vi "Write Variant Page Data.vi"(0 "Byte Stream File in":refnum<file>, 2 "Details":T2 {"PhotometricInterpretation" items=["MIN IS WHITE"=0, "MIN IS BLACK"=1, "RGB"=2, "PALETTE"=3, "MASK"=4, "SEPARATED"=5, "YCBCR"=6, "CIE LAB"=8, "ICC LAB"=9, "ITU LAB"=10, "LOGL"=32844, "LOGLUV"=32845, "CFA"=32803, "LinearRaw"=34892, "DEPTH"=51177]}, 5 "byte order (0:big-endian, network order)":T3(ring), 9 "Image Data":variant, 11 "error in (no error)":errorcluster, 13 "Settings":T1={"zlib compression level"=-1, "Max Strip bytes"=8192, "JPEG Quality (85)"=85}) -> (1 "Size(s)":u32[](array[numeric]), 3 "Bits per Sample":u32, 4 "Byte Stream File out":refnum<file>, 6 "Signed":bool, 8 "Data Bytes":i64, 10 "Bytes Per Sample":u32, 12 "Fractional":bool, 14 "Samples Per Pixel":i32, 15 "error out":errorcluster)   [LabVIEW 2020, in "LV Tiff.lvlib"]
uses:
  LV Tiff.lvlib
  Tiff Page Details.ctl
  Page Writer Settings.ctl
  <vilib>/picture/picture.llb/imagedata.ctl
  <vilib>/Utility/Data Type/NI_Data Type.lvlib
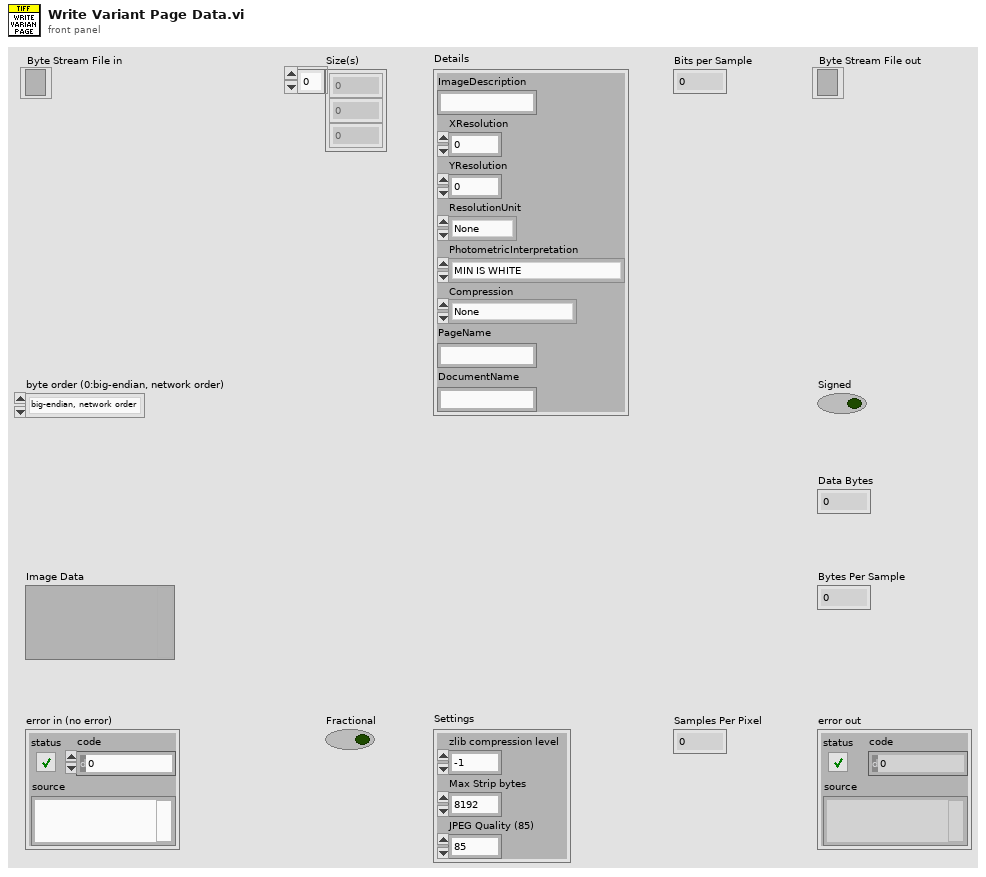
[diagram p1: front panel]
types:
  T1 = typedef "LV Tiff.lvlib/Page Writer Settings.ctl" = cluster{"zlib compression level":i32, "Max Strip bytes":u32, "JPEG Quality (85)":i32}
  T2 = typedef "LV Tiff.lvlib/Tiff Page Details.ctl" = cluster{"ImageDescription":string, "XResolution":dbl, "YResolution":dbl, "ResolutionUnit":enum16{"None", "Inch", "Centimeter"}, "PhotometricInterpretation":u16, "Compression":enum16{"None", "Deflate", "JPEG"}, "PageName":string, "DocumentName":string}
  T3 = enum16{"big-endian, network order", "native, host order", "little-endian"}
  T4 = typedef "imagedata.ctl" = cluster{"image type":i32, "image depth":i32, "image":u8[], "mask":u8[], "colors":u32[], "Rectangle":cluster{"left":i16, "top":i16, "right":i16, "bottom":i16}}
  T5 = typedef "NI_Data Type.lvlib/Data Type.ctl" = enum8{"Invalid Type", "Void", "I8", "I16", "I32", "I64", "U8", "U16", "U32", "U64", "Single Float", "Double Float", "Extended Float", "Single Complex", "Double Complex", "Extended Complex", "Enum U8", "Enum U16", "Enum U32", "Enum U64", "Single Float With Unit", "Double Float With Unit", "Extended Float With Unit", "Single Complex with Unit", "Double Complex with Unit", "Extended Complex with Unit", "Boolean", "String", "Path", "Picture", "Tag", "Array", "Cluster", "Variant", "LV Variant", "Waveform", "Timestamp", "Digital Waveform", "Digital Data", "ExpressData", "Refnum", "External Data", "VI", "Poly VI", "LabVIEW Class Instance", "Fixed Point", "Set Collection", "Map Collection"}
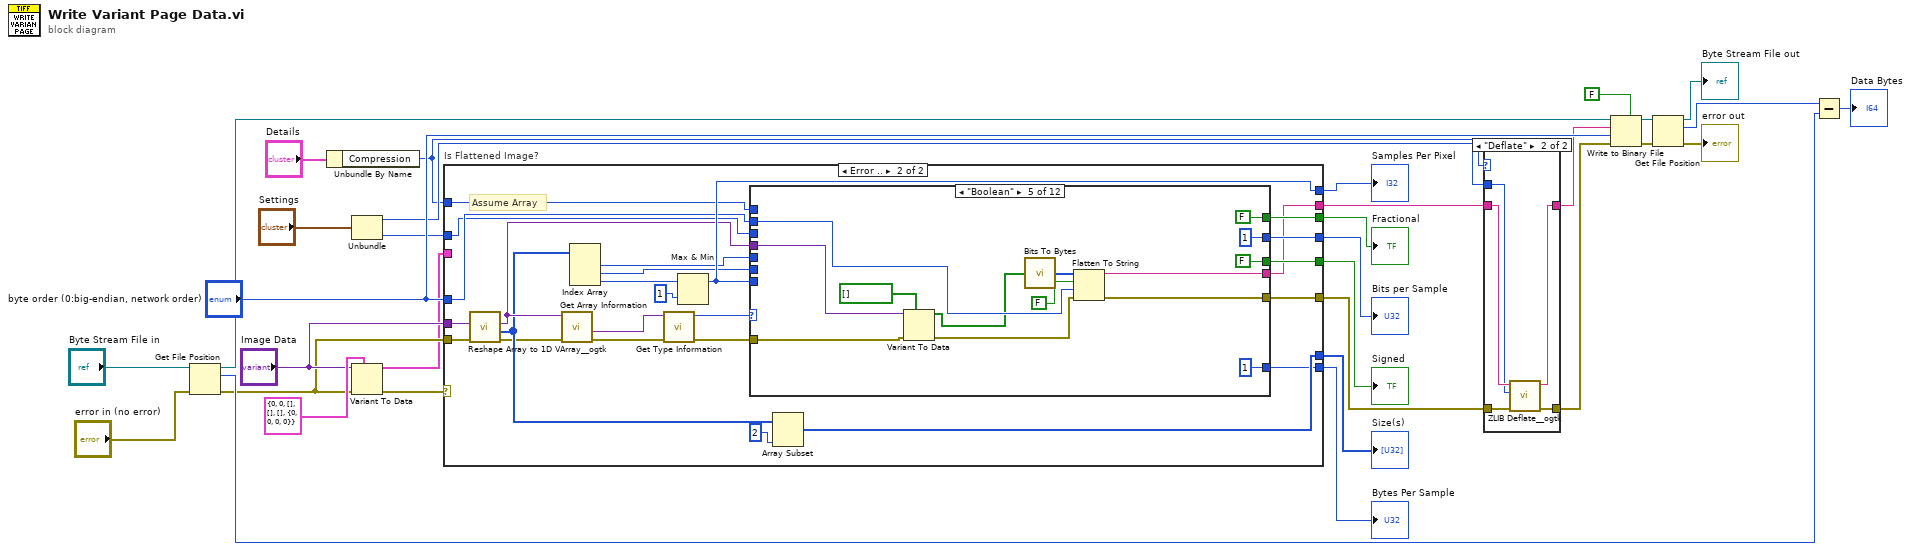
[diagram p0: block diagram]
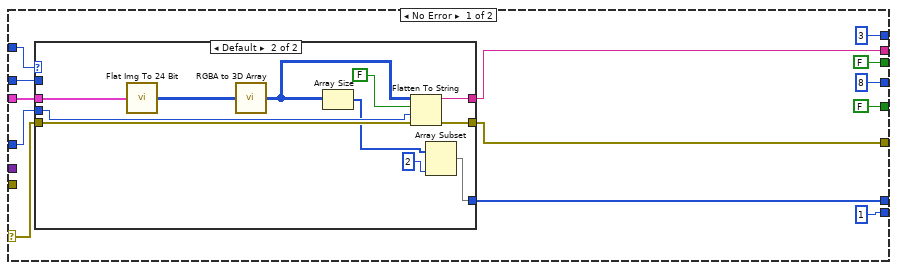
[diagram p2: hidden frame]
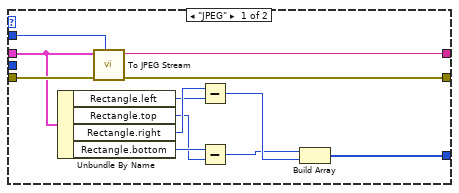
[diagram p3: hidden frame]
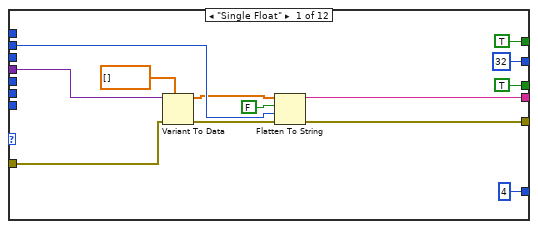
[diagram p4: hidden frame]
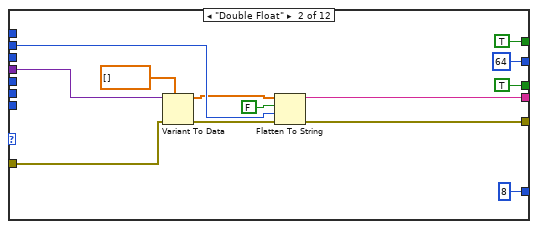
[diagram p5: hidden frame]
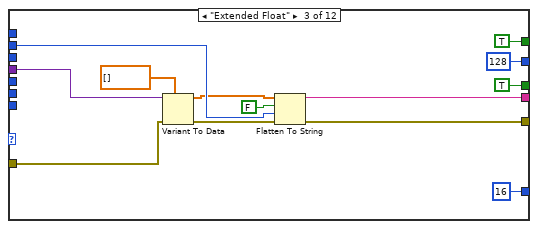
[diagram p6: hidden frame]
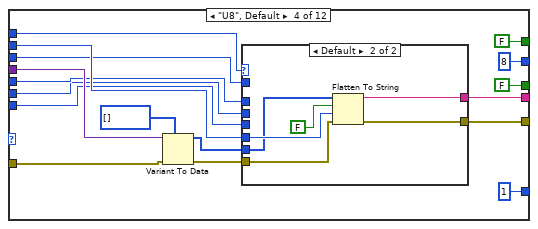
[diagram p7: hidden frame]
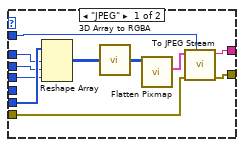
[diagram p8: hidden frame]
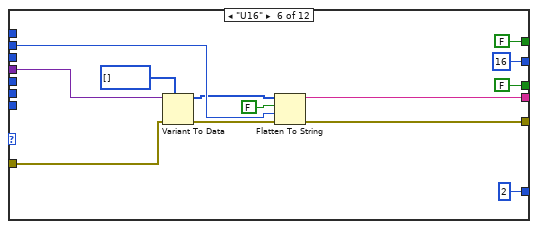
[diagram p9: hidden frame]
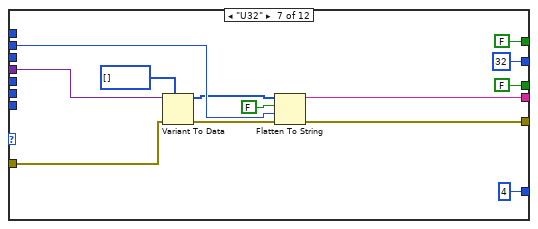
[diagram p10: hidden frame]
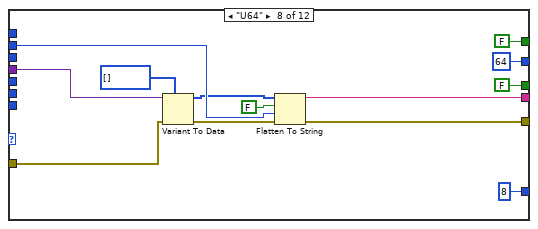
[diagram p11: hidden frame]
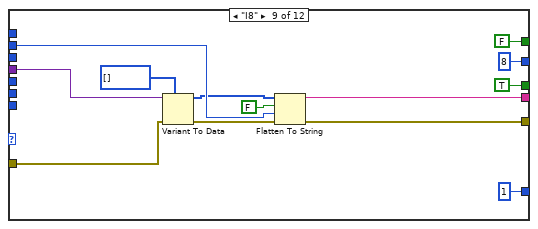
[diagram p12: hidden frame]
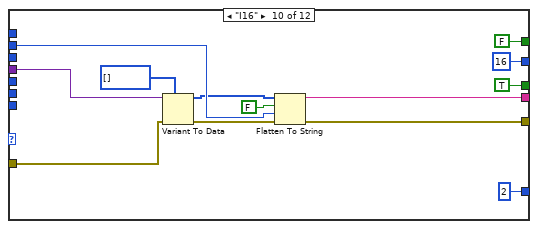
[diagram p13: hidden frame]
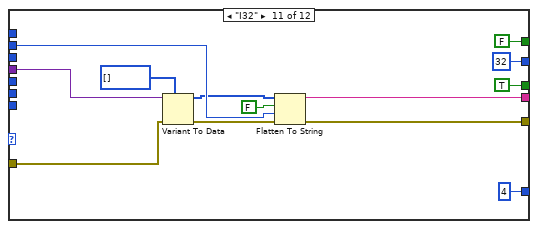
[diagram p14: hidden frame]
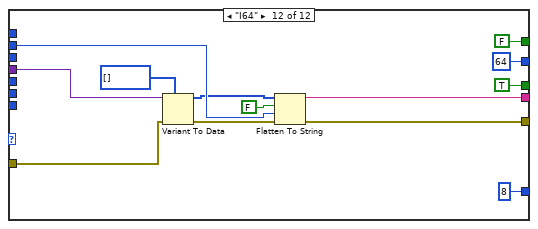
[diagram p15: hidden frame]
diagram:
  n1 = Get File Position(4:"error in (no error)", 7:"Byte Stream File in") -> (0:w4:errorcluster, 2:w17:i64, 3:w19:refnum<file>)
  n2 = Unbundle By Name("Details") -> ("Compression"=w7:enum16{"None", "Deflate", "JPEG"})
  n3 = Unbundle("Settings") -> ("zlib compression level"=w8:i32, "JPEG Quality (85)"=w1:i32)  [unwired: 1 out]
  n4 = Variant To Data(error in=w4, type=T4 {"image type"=0, "image depth"=0, "image"=[], "mask"=[], "colors"=[], "Rectangle"={"left"=0, "top"=0, "right"=0, "bottom"=0}} ("image data"), Variant="Image Data") -> (data=w2:T4, error out=w3:errorcluster)
  n5 = case "Is Flattened Image?" shown="Error .." w3 {
    selector: w3 -> [w38 _]
    tunnel: [u32 3 w93] -> w32
    tunnel: [w35 w92] -> w30
    tunnel: [u32 8 w91] -> w29
    tunnel: [u32 1 w90] -> w28
    tunnel: [FALSE w89] -> w27
    tunnel: [FALSE w88] -> w26
    tunnel: "byte order (0:big-endian, network order)" -> [w39 w87]
    tunnel: w4 -> [_ w74]
    tunnel: [w36 w73] -> w13
    tunnel: [w37 w72] -> w12
    tunnel: w7 -> [w34 w71]
    tunnel: "Image Data" -> [_ w70]
    tunnel: w2 -> [w40 _]
    tunnel: w1 -> [w33 w69]
    frame No Error {
      n6 = case shown="Default" w34 {
        tunnel: w40 -> [w54 w68]
        tunnel: w39 -> [_ w67]
        tunnel: w38 -> [w57 w66]
        tunnel: [w55 w65] -> w37
        tunnel: [w56 w64] -> w36
        tunnel: [w47 w59] -> w35
        tunnel: w33 -> [w46 _]
        frame "JPEG" {
          n7 = Unbundle By Name(w54) -> ("Rectangle.left"=w52:i16, "Rectangle.top"=w50:i16, "Rectangle.right"=w53:i16, "Rectangle.bottom"=w51:i16)
          n8 = call "To JPEG Stream.vi"("Quality (85)"=w46, "error out"=w57, "image data"=w54) -> ("error out"=w56:errorcluster, "data"=w55:string)  [unwired: 7 in]
          n9 = Subtract(x=w53, y=w52) -> (x-y=w49:i16)
          n10 = Subtract(x=w51, y=w50) -> (x-y=w48:i16)
          n11 = Build Array(w48, w49) -> (w47:i16[])
        }
        frame Default {
          n12 = call "Flat Img To 24 Bit.vi"("image data"=w68) -> ("24-bit pixmap"=w62:u32[][])
          n13 = call "RGBA to 3D Array.vi"("24-bit pixmap"=w62) -> ("RGB Array"=w60:u8[][][])  [unwired: 1 in]
          n14 = Array Size(array=w60) -> (size(s)=w61:i32[])
          n15 = Flatten To String(anything=w60, prepend array or string size? (T)=FALSE, byte order (0:big-endian, network order)=w67, error in (no error)=w66) -> (data string=w65:string, error out=w64:errorcluster)  [unwired: 1 out]
          n16 = Array Subset(array=w61, length=2) -> (w59:i32[])  [unwired: 1 in]
        }
      }
    }
    frame Error {
      # "Assume Array"
      n17 = call <userlib>:"Reshape Array to 1D VArray__ogtk.vi"("error in (no error)"=w74, "MultiD Array"=w70) -> ("error out"=w78:errorcluster, "Size(s)"=w80:u32[], "1D VArray"=w82:variant)  [unwired: 7 in]
      n18 = call <vilib>:"Get Array Information.vi"("error in (no error)"=w78, "variant"=w82) -> ("error out"=w84:errorcluster, "array element data type"=w83:variant)  [unwired: 6 in, 2 out]
      n19 = Index Array(array=w80) -> (element #1=w76:u32, element #2=w75:u32, element #3=w77:u32)  [unwired: 3 in]
      n20 = call <vilib>:"Get Type Information.vi"("error in (no error)"=w84, "variant"=w83) -> ("error out"=w86:errorcluster, "type"=w85:T5)  [unwired: 5 in, 3 out]
      n21 = Max & Min(x=w77, y=u32 1) -> (max(x,y)=w93:u32)  [unwired: 1 out]
      n22 = case shown="\"Boolean\"" w85 {
        tunnel: w87 -> [w105 w118 w131 w148 w179 w192 w205 w218 w231 w244 w257 w270]
        tunnel: [w104 w117 w130 w149 w180 w191 w204 w217 w230 w243 w256 w269] -> w73
        tunnel: [TRUE ("Signed") TRUE ("Signed") TRUE ("Signed") FALSE ("Signed") FALSE ("Signed") FALSE ("Signed") FALSE ("Signed") FALSE ("Signed") TRUE ("Signed") TRUE ("Signed") TRUE ("Signed") TRUE ("Signed")] -> w88
        tunnel: [TRUE ("Fractional") TRUE ("Fractional") TRUE ("Fractional") FALSE ("Fractional") FALSE ("Fractional") FALSE ("Fractional") FALSE ("Fractional") FALSE ("Fractional") FALSE ("Fractional") FALSE ("Fractional") FALSE ("Fractional") FALSE ("Fractional")] -> w89
        tunnel: [4 ("#Bytes") 8 ("#Bytes") 16 ("#Bytes") 1 ("#Bytes") 1 ("#Bytes") 2 ("#Bytes") 4 ("#Bytes") 8 ("#Bytes") 1 ("#Bytes") 2 ("#Bytes") 4 ("#Bytes") 8 ("#Bytes")] -> w90
        tunnel: [32 ("# Bits") 64 ("# Bits") 128 ("# Bits") 8 ("# Bits") 1 ("# Bits") 16 ("# Bits") 32 ("# Bits") 64 ("# Bits") 8 ("# Bits") 16 ("# Bits") 32 ("# Bits") 64 ("# Bits")] -> w91
        tunnel: w86 -> [w103 w116 w129 w145 w177 w190 w203 w216 w229 w242 w255 w268]
        tunnel: w82 -> [w102 w115 w128 w144 w176 w189 w202 w215 w228 w241 w254 w267]
        tunnel: w76 -> [_ _ _ w140 _ _ _ _ _ _ _ _]
        tunnel: w75 -> [_ _ _ w139 _ _ _ _ _ _ _ _]
        tunnel: w93 -> [_ _ _ w138 _ _ _ _ _ _ _ _]
        tunnel: [w94 w107 w120 w147 w178 w181 w194 w207 w220 w233 w246 w259] -> w72
        tunnel: w71 -> [_ _ _ w146 _ _ _ _ _ _ _ _]
        tunnel: w69 -> [_ _ _ w133 _ _ _ _ _ _ _ _]
        frame "Single Float" {
          n23 = Variant To Data(error in=w103, type=sgl[] [], Variant=w102) -> (data=w95:sgl[], error out=w100:errorcluster)
          n24 = Flatten To String(anything=w95, prepend array or string size? (T)=FALSE, byte order (0:big-endian, network order)=w105, error in (no error)=w100) -> (data string=w94:string, error out=w104:errorcluster)  [unwired: 1 out]
        }
        frame "Double Float" {
          n25 = Variant To Data(error in=w116, type=dbl[] [], Variant=w115) -> (data=w113:dbl[], error out=w112:errorcluster)
          n26 = Flatten To String(anything=w113, prepend array or string size? (T)=FALSE, byte order (0:big-endian, network order)=w118, error in (no error)=w112) -> (data string=w107:string, error out=w117:errorcluster)  [unwired: 1 out]
        }
        frame "Extended Float" {
          n27 = Variant To Data(error in=w129, type=ext[] [], Variant=w128) -> (data=w126:ext[], error out=w125:errorcluster)
          n28 = Flatten To String(anything=w126, prepend array or string size? (T)=FALSE, byte order (0:big-endian, network order)=w131, error in (no error)=w125) -> (data string=w120:string, error out=w130:errorcluster)  [unwired: 1 out]
        }
        frame "U8", Default {
          n29 = Variant To Data(error in=w145, type=u8[] [], Variant=w144) -> (data=w141:u8[], error out=w142:errorcluster)
          n30 = case shown="Default" w146 {
            tunnel: [w152 w166] -> w149
            tunnel: w148 -> [_ w165]
            tunnel: [w151 w163] -> w147
            tunnel: w142 -> [w153 w162]
            tunnel: w141 -> [w160 w161]
            tunnel: w140 -> [w159 _]
            tunnel: w139 -> [w158 _]
            tunnel: w138 -> [w157 _]
            tunnel: w133 -> [w150 _]
            frame "JPEG" {
              n31 = Reshape Array(w160, w159, w158, w157) -> (w156:u8[][][])
              n32 = call "3D Array to RGBA.vi"("3D Array"=w156) -> ("RGBA"=w155:u32[][])
              n33 = call <vilib>:"Flatten Pixmap.vi"("24-bit pixmap"=w155) -> ("image data"=w154:T4)  [unwired: 10 in]
              n34 = call "To JPEG Stream.vi"("Quality (85)"=w150, "error out"=w153, "image data"=w154) -> ("error out"=w152:errorcluster, "data"=w151:string)  [unwired: 7 in]
            }
            frame Default {
              n35 = Flatten To String(anything=w161, prepend array or string size? (T)=FALSE, byte order (0:big-endian, network order)=w165, error in (no error)=w162) -> (data string=w163:string, error out=w166:errorcluster)  [unwired: 1 out]
            }
          }
        }
        frame "Boolean" {
          n36 = Variant To Data(error in=w177, type=bool[] [], Variant=w176) -> (data=w173:bool[], error out=w174:errorcluster)
          n37 = call "Bits To Bytes.vi"("Bits"=w173) -> ("Bytes"=w167:u8[])
          n38 = Flatten To String(anything=w167, prepend array or string size? (T)=FALSE, byte order (0:big-endian, network order)=w179, error in (no error)=w174) -> (data string=w178:string, error out=w180:errorcluster)  [unwired: 1 out]
        }
        frame "U16" {
          n39 = Variant To Data(error in=w190, type=u16[] [], Variant=w189) -> (data=w187:u16[], error out=w186:errorcluster)
          n40 = Flatten To String(anything=w187, prepend array or string size? (T)=FALSE, byte order (0:big-endian, network order)=w192, error in (no error)=w186) -> (data string=w181:string, error out=w191:errorcluster)  [unwired: 1 out]
        }
        frame "U32" {
          n41 = Variant To Data(error in=w203, type=u32[] [], Variant=w202) -> (data=w200:u32[], error out=w199:errorcluster)
          n42 = Flatten To String(anything=w200, prepend array or string size? (T)=FALSE, byte order (0:big-endian, network order)=w205, error in (no error)=w199) -> (data string=w194:string, error out=w204:errorcluster)  [unwired: 1 out]
        }
        frame "U64" {
          n43 = Variant To Data(error in=w216, type=u64[] [], Variant=w215) -> (data=w213:u64[], error out=w212:errorcluster)
          n44 = Flatten To String(anything=w213, prepend array or string size? (T)=FALSE, byte order (0:big-endian, network order)=w218, error in (no error)=w212) -> (data string=w207:string, error out=w217:errorcluster)  [unwired: 1 out]
        }
        frame "I8" {
          n45 = Variant To Data(error in=w229, type=i8[] [], Variant=w228) -> (data=w226:i8[], error out=w225:errorcluster)
          n46 = Flatten To String(anything=w226, prepend array or string size? (T)=FALSE, byte order (0:big-endian, network order)=w231, error in (no error)=w225) -> (data string=w220:string, error out=w230:errorcluster)  [unwired: 1 out]
        }
        frame "I16" {
          n47 = Variant To Data(error in=w242, type=i16[] [], Variant=w241) -> (data=w239:i16[], error out=w238:errorcluster)
          n48 = Flatten To String(anything=w239, prepend array or string size? (T)=FALSE, byte order (0:big-endian, network order)=w244, error in (no error)=w238) -> (data string=w233:string, error out=w243:errorcluster)  [unwired: 1 out]
        }
        frame "I32" {
          n49 = Variant To Data(error in=w255, type=i32[] [], Variant=w254) -> (data=w252:i32[], error out=w251:errorcluster)
          n50 = Flatten To String(anything=w252, prepend array or string size? (T)=FALSE, byte order (0:big-endian, network order)=w257, error in (no error)=w251) -> (data string=w246:string, error out=w256:errorcluster)  [unwired: 1 out]
        }
        frame "I64" {
          n51 = Variant To Data(error in=w268, type=i64[] [], Variant=w267) -> (data=w265:i64[], error out=w264:errorcluster)
          n52 = Flatten To String(anything=w265, prepend array or string size? (T)=FALSE, byte order (0:big-endian, network order)=w270, error in (no error)=w264) -> (data string=w259:string, error out=w269:errorcluster)  [unwired: 1 out]
        }
      }
      n53 = Array Subset(array=w80, length=2) -> (w92:u32[])  [unwired: 1 in]
    }
  }
  "Samples Per Pixel" <- w32
  "Size(s)" <- w30
  "Bits per Sample" <- w29
  "Bytes Per Sample" <- w28
  "Fractional" <- w27
  "Signed" <- w26
  n54 = case shown="\"Deflate\"" w7 {
    tunnel: w13 -> [w273 w278]
    tunnel: w12 -> [w272 w277]
    tunnel: [w272 w276] -> w11
    tunnel: [w273 w275] -> w10
    tunnel: w8 -> [_ w274]
    frame Default {
    }
    frame "Deflate" {
      n55 = call <userlib>:"ZLIB Deflate__ogtk.vi"("error in (no error)"=w278, "compression level (default)"=w274, "input"=w277) -> ("error out"=w275:errorcluster, "deflated output"=w276:string)  [unwired: 2 in, 1 out]
    }
  }
  n56 = Write to Binary File(file (use dialog)=w19, data=w11, error in=w10, 5:FALSE ("prepend array or string size? (T)"), 9:"byte order (0:big-endian, network order)") -> (refnum out=w15:refnum<file>, error out=w14:errorcluster)  [unwired: 1 in, 1 out]
  n57 = Get File Position(4:w14, 7:w15) -> (0:→"error out":errorcluster, 2:w18:i64, 3:→"Byte Stream File out":refnum<file>)
  n58 = Subtract(x=w18, y=w17) -> (x-y=→"Data Bytes":i64)
